vi "solar_voy Write (Variant).vi"(4 "HDR_GUID":string, 5 "TARGET":string, 6 "Suppress Errors? (T)":bool=TRUE, 7 "CMD":enum8{"CMD", "TLM"}(ring), 8 "error in (no error)":errorcluster, 9 "Variant (No HDR)":variant, 10 "PACKET (\"\" = Use Variant)":string, 11 "Voyager Refnum in":T1) -> (0 "error out":errorcluster, 3 "Voyager Refnum out":T1)   [LabVIEW 2018]
doc: "This looks up and writes the packet by name. The Variant should not contain the header items. If <b>PACKET</b> is empty this uses the variant name as the packet name."
uses:
  solar_voy_ctl Voyager Refnum.ctl
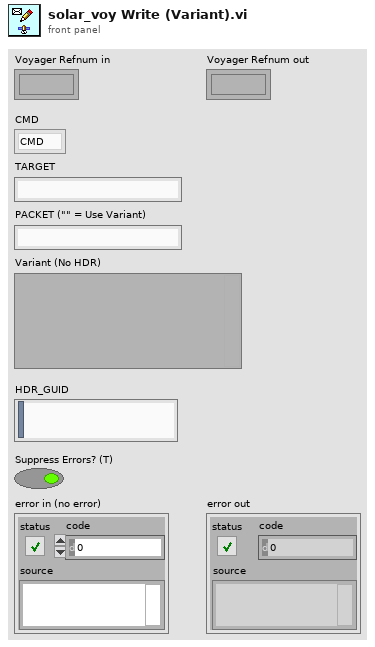
[diagram p1: front panel]
types:
  T1 = typedef "solar_voy_ctl Voyager Refnum.ctl" = refnum<k1>
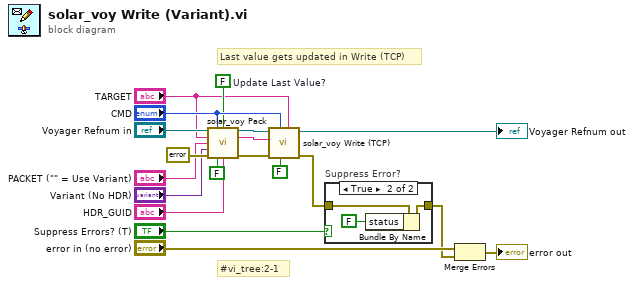
[diagram p0: block diagram]
diagram:
  w2 = FALSE  # Update Last Value?
  # "Last value gets updated in Write (TCP)"
  # "#vi_tree:2-1"
  n1 = call "solar_voy Pack.vi"("Voyager Refnum in"="Voyager Refnum in", "CMD"="CMD", "Update Last Value? (F)"=w2, "TARGET"="TARGET", "PACKET (\"\" = Use Variant)"="PACKET (\"\" = Use Variant)", "Variant (No HDR)"="Variant (No HDR)", "error in (no error)"=errorcluster {"status"=FALSE, "code"=0, "source"=""}, "Suppress Errors? (T)"=FALSE, "HDR_GUID"="HDR_GUID") -> ("Voyager Refnum out"=w9:T1, "TCP Data to Send"=w4:string, "error out"=w12:errorcluster)  [unwired: 3 in, 1 out]
  n2 = call "solar_voy Write (TCP).vi"("TARGET"="TARGET", "Suppress Errors? (T)"=FALSE, "CMD"="CMD", "error in (no error)"=w12, "TCP Data to Send"=w4, "Voyager Refnum in"=w9) -> ("error out"=w14:errorcluster, "Voyager Refnum out"=→"Voyager Refnum out":T1)  [unwired: 3 in, 1 out]
  n3 = case "Suppress Error?" shown="True" "Suppress Errors? (T)" {
    tunnel: w14 -> [w20 w23]
    tunnel: [w20 w22] -> w17
    frame False {
    }
    frame True {
      n4 = Bundle By Name(cluster=w23, "status"=FALSE) -> (w22:errorcluster)
    }
  }
  n5 = Merge Errors("error in (no error)", w17) -> (→"error out":errorcluster)
